vi "Load to Subpanel.vi"(0 "Sub Panel Ref In":refnum<vi>, 5 "VI Refs In":refnum<vi>[](array[refnum]), 7 "Module Name In":string, 11 "error in (no error)":errorcluster) -> (4 "Sub Panel Ref Out":refnum<vi>, 6 "VI Refs Out":refnum<vi>[](array[refnum]), 8 "Module Name Out":string, 15 "error out":errorcluster)   [LabVIEW 2019, in "Subpanel Tools.lvlib"]
doc: "This VI bring the Frontpanel to a Subpanel."
uses:
  Subpanel Tools.lvlib
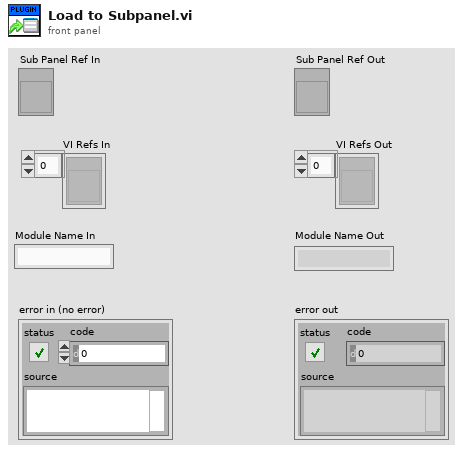
[diagram p1: front panel]
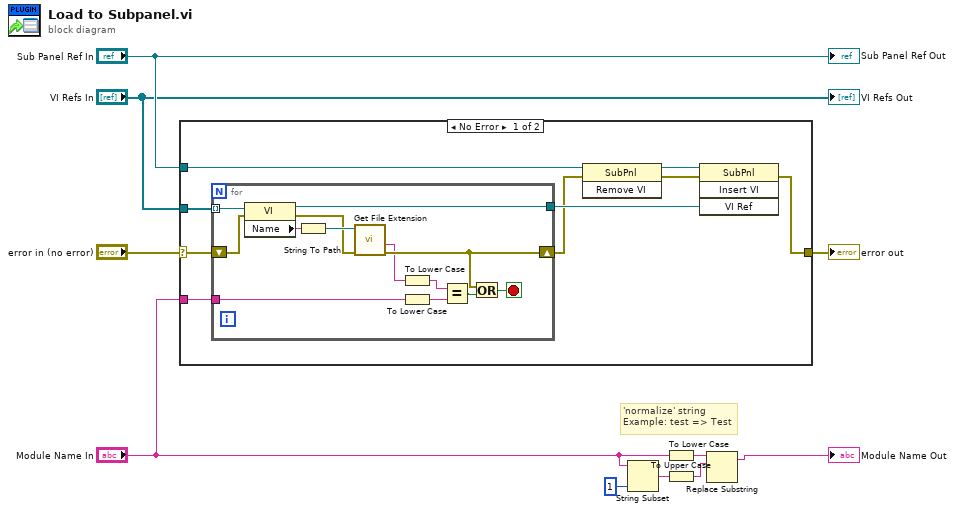
[diagram p0: block diagram]
diagram:
  # "'normalize' string\nExample: test => Test"
  n1 = case shown="No Error" "error in (no error)" {
    selector: "error in (no error)" -> [w14 w33]
    tunnel: "Module Name In" -> [w11 _]
    tunnel: [w15 w33] -> w10
    tunnel: "Sub Panel Ref In" -> [w13 _]
    tunnel: "VI Refs In" -> [w12 _]
    frame No Error {
      n2 = for {
        tunnel: w12 -> [w32] mode=indexing
        tunnel: w11 -> [w24]
        tunnel: [w27] -> w17
        shift-right: [w26] -> w16
        shift-left: w14 -> [w25]
        stop <- w28 stop-if-true
        n3 = property class="VI"(reference=w32, error in=w25) -> (reference out=w27:refnum<vi>, error out=w29:errorcluster, "Name"=w30:string)
        n4 = String To Path(string=w30) -> (path=w31:path)
        n5 = call <vilib>:"Get File Extension.vi"("error in (no error)"=w29, "file"=w31) -> ("error out"=w26:errorcluster, "filename without extension"=w23:string)  [unwired: 8 out]
        n6 = To Lower Case(string=w23) -> (all lower case string=w22:string)
        n7 = To Lower Case(string=w24) -> (all lower case string=w21:string)
        n8 = Equal?(x=w22, y=w21) -> (x = y?=w20:bool)
        n9 = Or(x=w26, y=w20) -> (x .or. y?=w28:bool)
      }
      n10 = invoke class="SubPnl" method="Remove VI"(reference=w13, error in=w16) -> (reference out=w19:refnum<vi>, error out=w18:errorcluster)  [unwired: 1 in, 1 out]
      n11 = invoke class="SubPnl" method="Insert VI"(reference=w19, error in=w18, "VI Ref"=w17) -> (error out=w15:errorcluster)  [unwired: 1 in, 3 out]
    }
    frame Error {
    }
  }
  "error out" <- w10
  n12 = String Subset(string="Module Name In", length (rest)=1 ("length (rest)")) -> (substring=w4:string)  [unwired: 1 in]
  n13 = To Lower Case(string="Module Name In") -> (all lower case string=w5:string)
  n14 = To Upper Case(1:w4) -> (0:w3:string)
  n15 = Replace Substring(4:w3, 5:w5) -> (1:→"Module Name Out":string)  [unwired: 2 in, 1 out]
  "Sub Panel Ref Out" <- "Sub Panel Ref In"
  "VI Refs Out" <- "VI Refs In"
